vi "Post-Launch Initialize.vi"(8 "error in":errorcluster, 10 "GUI_Ref":refnum<vi>, 11 "Report Viewer in":refnum<class "Report Viewer.lvclass">) -> (0 "error out":errorcluster, 3 "Report Viewer out":refnum<class "Report Viewer.lvclass">, 4 "Registered Events":T1, 6 "Self Enqueuer":refnum<class "Message Enqueuer.lvclass">)   [LabVIEW 2019]
uses:
  Library/Report Viewer.lvclass
  builds/Engine/Panel.lvlibp/Panel Helper/Events.ctl
  builds/Engine/Panel.lvlibp/Panel Helper/Panel Events.ctl
  builds/Engine/Engine.lvlibp/Custom Controls/System Status.ctl
  builds/Engine/Engine.lvlibp/Custom Controls/System Events.ctl
  builds/Engine/Engine.lvlibp/Custom Controls/Manual Events.ctl
  builds/Engine/Engine.lvlibp/Custom Controls/UUT_Events.ctl
  builds/Engine/Engine.lvlibp/Custom Controls/Engine Events.ctl
  builds/Engine/Actor Framework.lvlibp/1abvi3w/vi.lib/ActorFramework/Message Enqueuer/Message Enqueuer.lvclass
  builds/Engine/Engine.lvlibp/Custom Controls/Interface Events.ctl
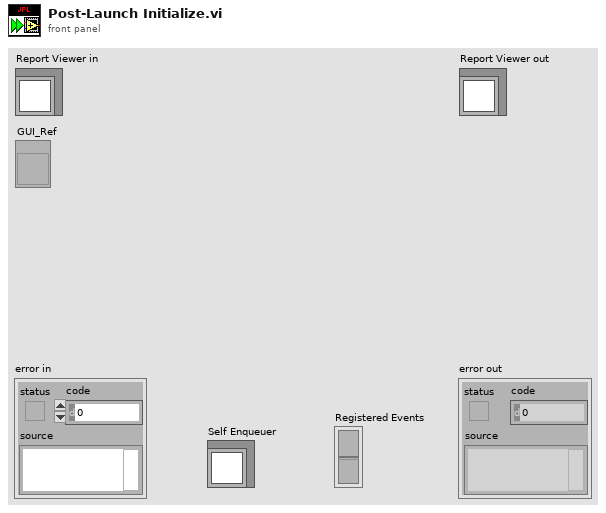
[diagram p1: front panel]
types:
  T1 = cluster{"Pnl Actor":refnum<event-registration>, "Event Registration Refnum":refnum<event-registration>}
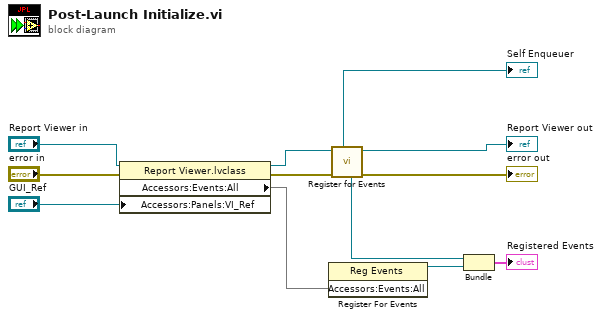
[diagram p0: block diagram]
diagram:
  n1 = property class="Report Viewer.lvclass"(reference="Report Viewer in", error in="error in", "Accessors:Panels:VI_Ref"="GUI_Ref") -> (reference out=w10:refnum<class "Report Viewer.lvclass">, error out=w12:errorcluster, "Accessors:Events:All"=w8)
  n2 = register-events(w8) -> (reference out=w7:refnum<event-registration>)  [unwired: 2 in, 1 out]
  n3 = call "Register for Events.vi"("Error In"=w12, "Panel Actor in"=w10) -> ("Error Out"=→"error out":errorcluster, "Panel Actor out"=→"Report Viewer out":refnum<class "Report Viewer.lvclass">, "Pnl Actor"=w9:refnum<event-registration>, "Self Enqueuer"=→"Self Enqueuer":refnum<class "Message Enqueuer.lvclass">)  [unwired: 6 in]
  n4 = Bundle("Pnl Actor"=w9, "Event Registration Refnum"=w7) -> (→"Registered Events":T1)  [unwired: 1 in]
